vi "On Message.vi"(8 "error in (no error)":errorcluster, 10 "Actor in":refnum<class "Actor.lvclass">, 11 "Client Connection Handler Msg in":refnum<class "Server Connection Handler Msg.lvclass">) -> (0 "error out":errorcluster, 2 "Actor out":refnum<class "Actor.lvclass">, 3 "Client Connection Handler Msg out":refnum<class "Server Connection Handler Msg.lvclass">)   [LabVIEW 2021, in "Echo Broadcast Test With Server Manager.lvlib" / "Server Connection Handler Msg.lvclass"]
uses:
  Server Connection Handler Msg.lvclass
  C:/Projects/WebSocket-Actor/WebSocket Actor/Abstract Messages/WebSocket Connection Handler Msg/WebSocket Connection Handler Msg.lvclass
  <vilib>/ActorFramework/Actor/Actor.lvclass
  WebSocket Actor/Abstract Messages/WebSocket Connection Handler Msg/WebSocket Connection Handler Msg.lvclass/WebSocket Connection Handler Msg.ctl
  WebSocket Actor/Abstract Messages/WebSocket Connection Handler Msg/properties/Read Connection Enqueuer.vi
  WebSocket Actor/Abstract Messages/WebSocket Connection Handler Msg/properties/Read Peer ID.vi
  WebSocket Actor/Abstract Messages/WebSocket Connection Handler Msg/properties/Read Data.vi
  <vilib>/ActorFramework/Message Enqueuer/Message Enqueuer.lvclass
  Server Connection Handler Msg.lvclass/Server Connection Handler Msg.ctl
  WebSocket Actor/WebSocket Service Messages/Send Msg/Send Msg.lvclass
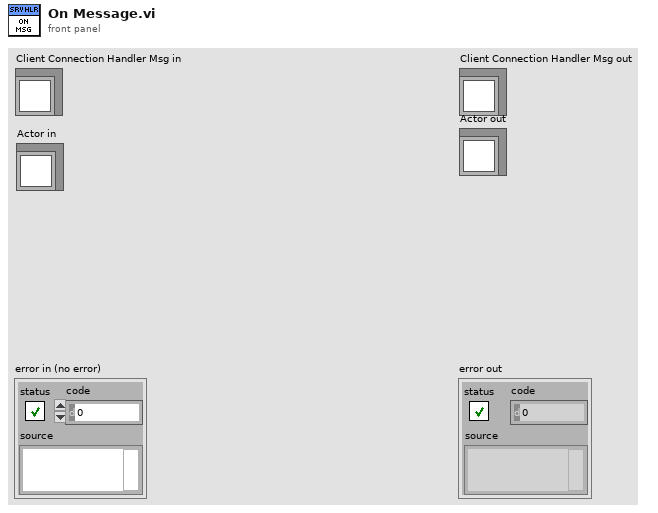
[diagram p1: front panel]
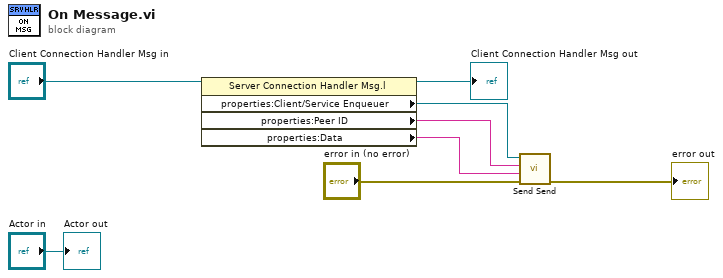
[diagram p0: block diagram]
diagram:
  n1 = property class="Server Connection Handler Msg.l"(reference="Client Connection Handler Msg in") -> (reference out=→"Client Connection Handler Msg out":refnum<class "Server Connection Handler Msg.lvclass">, "properties:Client/Service Enqueuer"=w5:refnum<class "Message Enqueuer.lvclass">, "properties:Peer ID"=w1:string, "properties:Data"=w3:string)  [unwired: 1 in, 1 out]
  n2 = call "Send Send.vi"("error in (no error)"="error in (no error)", "Data"=w3, "Client ID"=w1, "Message Enqueuer in"=w5) -> ("error out"=→"error out":errorcluster)  [unwired: 6 in, 1 out]
  "Actor out" <- "Actor in"
